vi "Insert Jump Step.vi"(0 "VISA resource name":refnum<visa-resource-name>, 1 "Unit Address (1)":i16=1, 2 "Jump To Profile Number (1)":i16=1, 5 "Current Step Number (1)":i16=1, 7 "Step Number (1)":i16=1, 9 "Number Of Repeats (1)":i16=1, 11 "error in (no error)":errorcluster {"code" format="%.0x"}) -> (4 "VISA resource name out":refnum<visa-resource-name>, 15 "error out":errorcluster {"code" format="%.0x"})   [LabVIEW 2010]
doc: "This VI inserts the Jump Step."
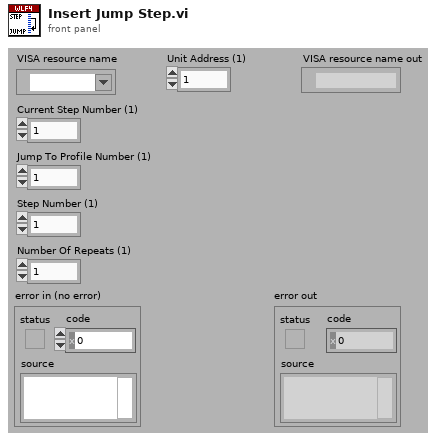
[diagram p1: front panel]
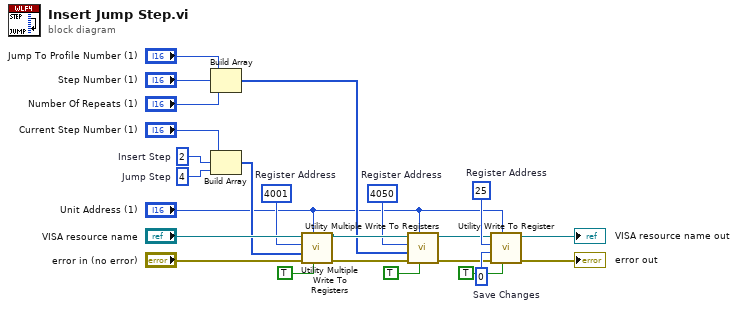
[diagram p0: block diagram]
diagram:
  w11 = u16 4050  # Register Address
  w15 = u16 2  # Insert Step
  w16 = i16 0  # Save Changes
  w17 = u16 25  # Register Address
  w20 = u16 4  # Jump Step
  w22 = u16 4001  # Register Address
  n1 = Build Array("Jump To Profile Number (1)", "Step Number (1)", "Number Of Repeats (1)") -> (w9:i16[])
  n2 = Build Array("Current Step Number (1)", w15, w20) -> (w21:u16[])
  n3 = call "Utility Multiple Write To Registers.vi"("Direct Action?"=TRUE, "Unit Address (1)"="Unit Address (1)", "error in (no error)"="error in (no error)", "Array Of Data"=w21, "Register Address (0)"=w22, "VISA resource name"="VISA resource name") -> ("error out"=w13:errorcluster, "VISA resource name out"=w12:refnum<visa-resource-name>)  [unwired: 4 in]
  n4 = call "Utility Multiple Write To Registers.vi"("Direct Action?"=TRUE, "Unit Address (1)"="Unit Address (1)", "error in (no error)"=w13, "Array Of Data"=w9, "Register Address (0)"=w11, "VISA resource name"=w12) -> ("error out"=w8:errorcluster, "VISA resource name out"=w7:refnum<visa-resource-name>)  [unwired: 4 in]
  n5 = call "Utility Write To Register.vi"("Direct Action?"=TRUE, "Unit Address (1)"="Unit Address (1)", "error in (no error)"=w8, "Data (0)"=w16, "Register Address (0)"=w17, "VISA resource name"=w7) -> ("error out"=→"error out":errorcluster, "VISA resource name out"=→"VISA resource name out":refnum<visa-resource-name>)  [unwired: 4 in]
